vi "Get_Shortcut.vi"(8 "error in (no error)":errorcluster, 11 "Class in":refnum<class "IB_Shortcut.lvclass">) -> (0 "error out":errorcluster, 2 "data":T1, 3 "Class out":refnum<class "IB_Shortcut.lvclass">)   [LabVIEW 2020, in "IB_Shortcut.lvclass"]
uses:
  <vilib>/AppBuilder/IB_Classes/Shortcut/IB_Shortcut.lvclass
  <vilib>/AppBuilder/IB_Classes/Shortcut/IB_Shortcut.lvclass/IB_Shortcut.ctl
  <vilib>/AppBuilder/IB_Classes/Shortcut/IB_Shortcut.ctl
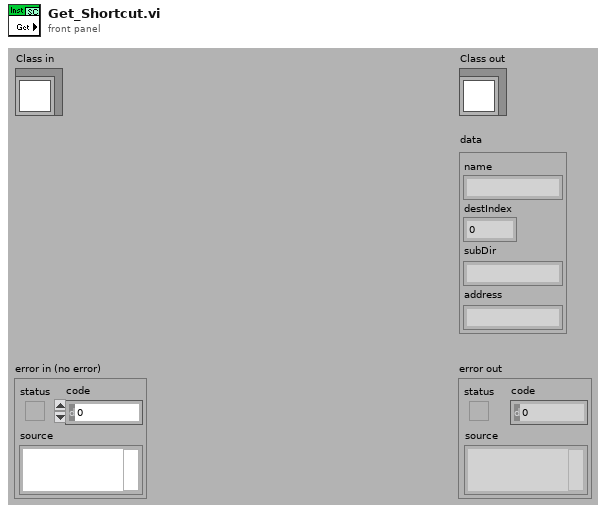
[diagram p1: front panel]
types:
  T1 = typedef "IB_Shortcut.ctl" = cluster{"name":string, "destIndex":i32, "subDir":string, "address":string}
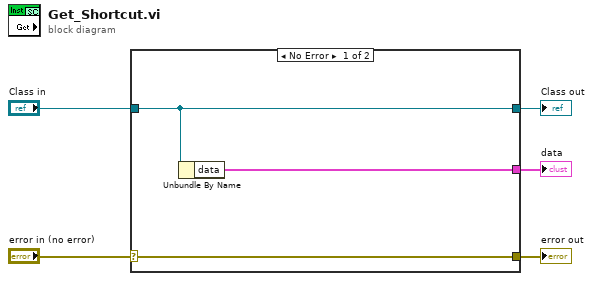
[diagram p0: block diagram]
diagram:
  n1 = case shown="No Error" "error in (no error)" {
    selector: "error in (no error)" -> [w8 w9]
    tunnel: [w8 w9] -> w4
    tunnel: [w7 w10] -> w2
    tunnel: "Class in" -> [w7 w10]
    tunnel: [w6 _] -> w1
    frame No Error {
      n2 = Unbundle By Name(w7) -> ("data"=w6:T1)
    }
    frame Error {
    }
  }
  "error out" <- w4
  "Class out" <- w2
  "data" <- w1
